vi "Get BC Scanner Info.vi"(0 "Prompt":string) -> (2 "Info Out":string, 4 "OK":bool)   [LabVIEW 2026]
panel:
  in  "Cancel":bool
  in  "Info In:":string
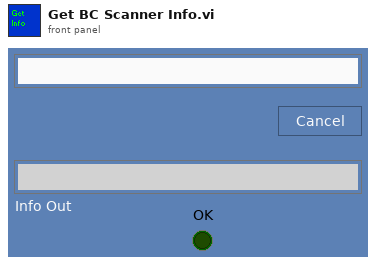
[diagram p1: front panel]
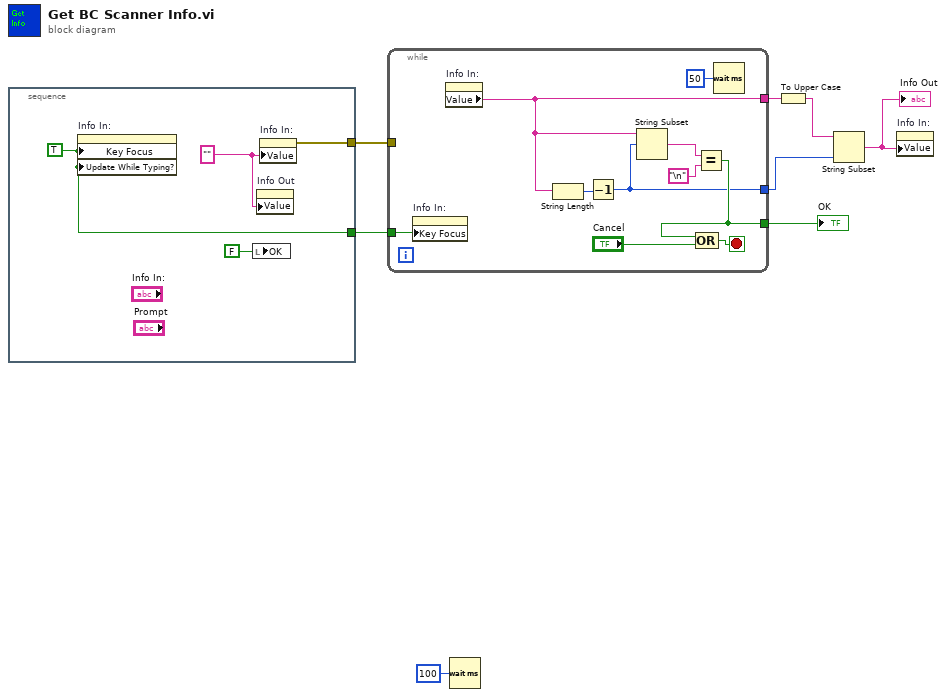
[diagram p0: block diagram]
diagram:
  n1 = stacked-sequence {
    tunnel: [w12] -> w5
    tunnel: [w9] -> w1
    frame #0 {
      w9 = TRUE ("Key Focus")
      w11 = "" ("Case Number:")
      n2 = property on="Info In:" class="Str"("Key Focus"=w9, "Update While Typing?"=w9) -> ()  [unwired: 2 in, 2 out]
      n3 = local write "OK"(FALSE ("OK")) -> ()
      n4 = property on="Info Out" class="Str"("Value"=w11) -> ()  [unwired: 2 in, 2 out]
      n5 = property on="Info In:" class="Str"("Value"=w11) -> (error out=w12:errorcluster)  [unwired: 2 in, 1 out]
    }
  }
  n6 = while {
    tunnel: [w14] -> w7
    tunnel: [w16] -> w8
    tunnel: w5 -> [_]
    tunnel: [w15] -> w3
    tunnel: w1 -> [w13]
    stop <- w21 stop-if-true
    n7 = property on="Info In:" class="Str"("Key Focus"=w13) -> ()  [unwired: 2 in, 2 out]
    n8 = property on="Info In:" class="Str"() -> ("Value"=w14:string)  [unwired: 2 in, 2 out]
    n9 = String Length(string=w14) -> (length=w19:i32)
    n10 = Decrement(x=w19) -> (x-1=w15:i32)
    n11 = String Subset(string=w14, offset (0)=w15) -> (substring=w18:string)  [unwired: 1 in]
    n12 = Equal?(x=w18, y="\n") -> (x = y?=w16:bool)
    n13 = Compound Arithmetic op=OR(w16, "Cancel") -> (w21:bool)
    n14 = Wait (ms)(milliseconds to wait=u32 50) -> ()  [unwired: 1 out]
  }
  "OK" <- w8
  n15 = Wait (ms)(milliseconds to wait=u32 100) -> ()  [unwired: 1 out]
  n16 = To Upper Case(1:w7) -> (0:w4:string)
  n17 = String Subset(string=w4, length (rest)=w3) -> (substring=w2:string)  [unwired: 1 in]
  "Info Out" <- w2
  n18 = property on="Info In:" class="Str"("Value"=w2) -> ()  [unwired: 2 in, 2 out]
